vi "Next.vi"(8 "error in (no error)":errorcluster, 11 "LUnit Test Suite In":refnum<class "LUnit Test Suite.lvclass">) -> (0 "error out":errorcluster, 1 "Suite":string, 2 "Name":string, 3 "LUnit Test Suite Out":refnum<class "LUnit Test Suite.lvclass">)   [LabVIEW 2020, in "LUnit Test Suite.lvclass"]
uses:
  LUnit Test Suite.lvclass
  LUnit Test Suite.lvclass/LUnit Test Suite.ctl
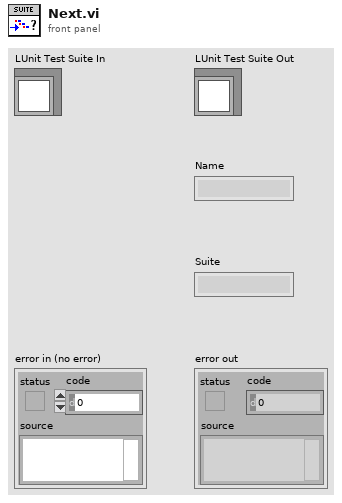
[diagram p1: front panel]
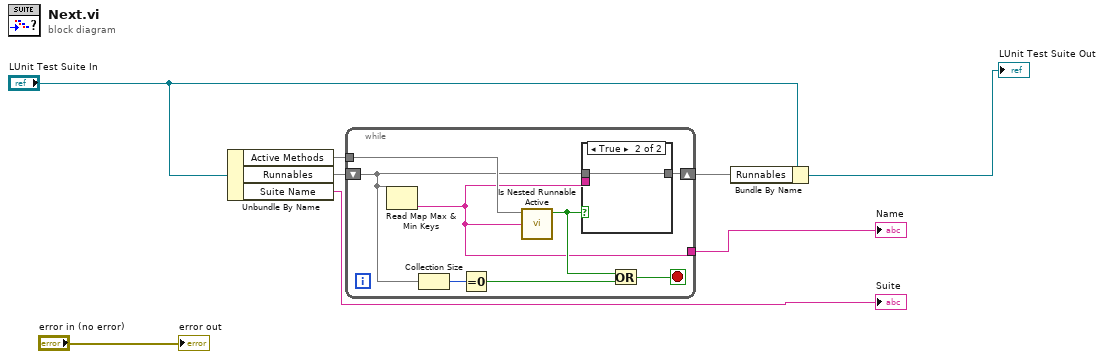
[diagram p0: block diagram]
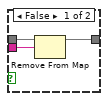
[diagram p2: hidden frame]
diagram:
  n1 = Unbundle By Name("LUnit Test Suite In") -> ("Active Methods"=w7:set{string}, "Runnables"=w8:map{string, refnum<class "Runnable.lvclass">}, "Suite Name"=→"Suite":string)
  n2 = while {
    tunnel: w7 -> [w16]
    shift-right: [w15] -> w6
    shift-left: w8 -> [w13]
    tunnel: [w9] -> w3
    stop <- w14 stop-if-true
    n3 = Read Map Max & Min Keys(11:w13) -> (1:w9:string)  [unwired: 1 out]
    n4 = Collection Size(1:w13) -> (0:w12:i32)
    n5 = Equal To 0?(x=w12) -> (x = 0?=w11:bool)
    n6 = call "Is Nested Runnable Active"("Name"=w9, "Active Methods"=w16) -> ("found?"=w10:bool)  [unwired: 9 in]
    n7 = case shown="True" w10 {
      tunnel: w9 -> [w19 _]
      tunnel: [w18 w20] -> w15
      tunnel: w13 -> [w17 w20]
      frame False {
        n8 = Remove From Map(10:w19, 11:w17) -> (3:w18:map{string, refnum<class "Runnable.lvclass">})  [unwired: 2 out]
      }
      frame True {
      }
    }
    n9 = Or(x=w10, y=w11) -> (x .or. y?=w14:bool)
  }
  "Name" <- w3
  n10 = Bundle By Name(cluster="LUnit Test Suite In", "Runnables"=w6) -> (→"LUnit Test Suite Out":refnum<class "LUnit Test Suite.lvclass">)
  "error out" <- "error in (no error)"
